vi "3.1-4.7.1-Act Client.vi"() -> ()   [LabVIEW 2010]
doc: "This is the act client, which should send hellos and wait for data. if it receives no data (times out) it continues sending hellos. if it fails in any other way, it closes the UDP connection and starts up a new one. The act control data type is strange because it contains a variant which is either joystick data or arbitratable data. an enumeration controls how it should be interpreted."
uses:
  4-High Neurons/4.0-Super Heart Beat.ctl
  4-High Neurons/4.1-Act Control Typedef.ctl
  4-High Neurons/4.1.0-Datatype Typedef.ctl
  4-High Neurons/4.1.1-Act Joystick.ctl
  4-High Neurons/4.1.2-Act Neuron TD.ctl
  3.0-Global.vi
panel:
  out "Super Heart Beat":T1
  out "Error":errorcluster
  in  "stop":bool
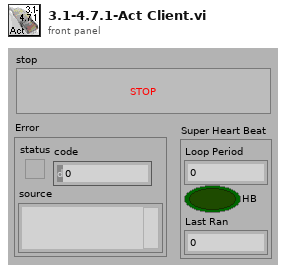
[diagram p1: front panel]
types:
  T1 = typedef "4.0-Super Heart Beat.ctl" = cluster{"Loop Period":u32, "HB":bool, "Last Ran":u32}
  T2 = typedef "4.1.1-Act Joystick.ctl" = cluster{"Trig":bool, "2":bool, "3":bool, "4":bool, "5":bool, "6":bool, "7":bool, "8":bool, "9":bool, "10":bool, "11":bool, "Pitch":i32, "Ang":bool[], "Wheel":dbl, "Roll":i32, "Yaw":i32, "Left":i32, "Right":i32}
  T3 = typedef "4.1.2-Act Neuron TD.ctl" = cluster{"Speed By Path":dbl[]}
  T4 = typedef "4.1-Act Control Typedef.ctl" = cluster{"4.1.0 Data":variant, "Type of Data":T5, "E-Stop":bool, "Restart":bool, "New IP":bool, "Begin":bool, "Time":i32, "Shutdown":bool}
  T5 = typedef "4.1.0-Datatype Typedef.ctl" = enum16{"4.1.0-Empty Data", "4.1.1-Joystick Data", "4.1.2-Behavioral Data"}
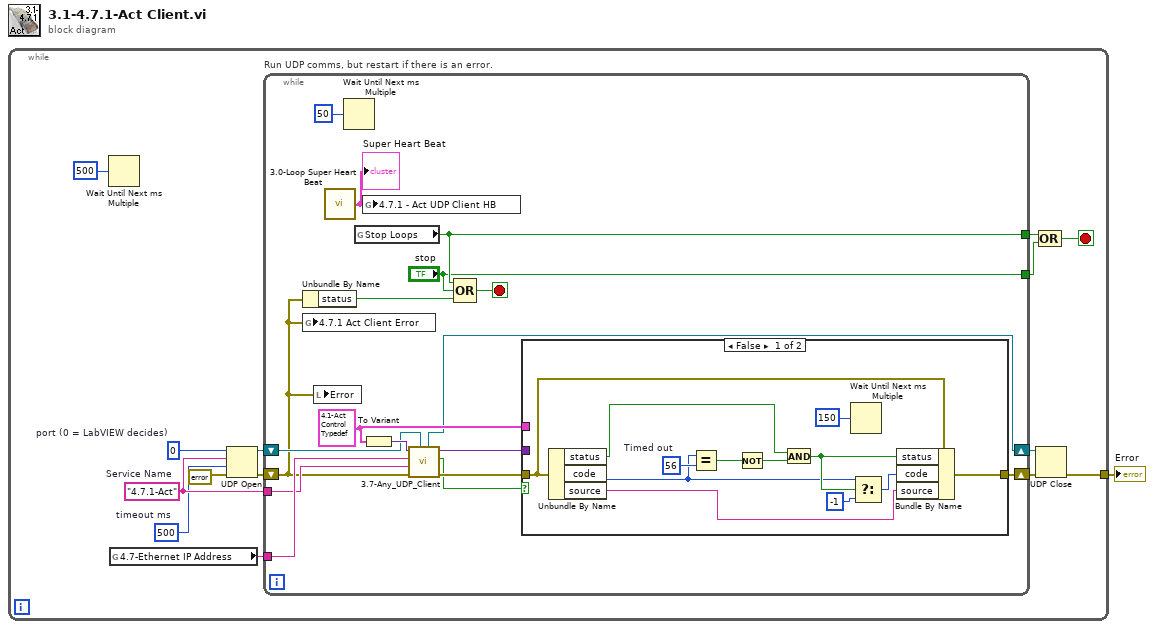
[diagram p0: block diagram]
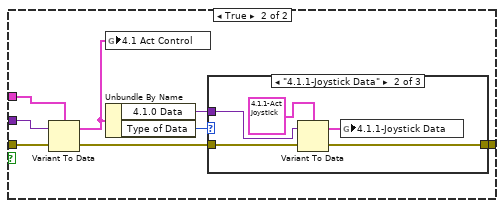
[diagram p2: hidden frame]
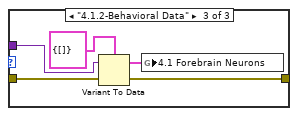
[diagram p4: hidden frame]
diagram:
  n1 = while {
    tunnel: [w3] -> w1
    stop <- w13 stop-if-true
    w6 = 500  # timeout ms
    w8 = u16 0  # port (0 = LabVIEW decides)
    w7 = "4.7.1-Act"  # Service Name
    n2 = Wait Until Next ms Multiple(millisecond multiple=u32 500) -> ()  [unwired: 1 out]
    n3 = global read "3.0-Global.vi" "4.7-Ethernet IP Address"() -> (w5:string)
    n4 = UDP Open(8:errorcluster {"status"=FALSE, "code"=0, "source"=""} ("error in (no error)"), 9:w6, 10:w7, 11:w8) -> (port=w12:refnum<k16>, 0:w10:errorcluster)  [unwired: 1 in, 1 out]
    n5 = while "Run UDP comms, but restart if there is an error." {
      tunnel: w7 -> [w29]
      tunnel: w5 -> [w30]
      tunnel: [w25] -> w15
      tunnel: ["stop"] -> w14
      shift-right: [w21] -> w11
      shift-left: w12 -> [w22]
      shift-right: [w20] -> w9
      shift-left: w10 -> [w17]
      stop <- w32 stop-if-true
      w26 = T4 {"4.1.0 Data"=variant, "Type of Data"=enum."4.1.1-Joystick Data", "E-Stop"=FALSE, "Restart"=FALSE, "New IP"=FALSE, "Begin"=FALSE, "Time"=0, "Shutdown"=FALSE} ("4.1 Act Control")
      n6 = Unbundle By Name(w17) -> ("status"=w23:bool)
      n7 = global write "3.0-Global.vi" "4.7.1 Act Client Error"(w17) -> ()
      n8 = local write "Error"(w17) -> ()
      n9 = call "3.0-Loop Super Heart Beat.vi"() -> ("Super Heart Beat"=w16:T1)
      "Super Heart Beat" <- w16
      n10 = Wait Until Next ms Multiple(millisecond multiple=u32 50) -> ()  [unwired: 1 out]
      n11 = global read "3.0-Global.vi" "Stop Loops"() -> (w25:bool)
      n12 = global write "3.0-Global.vi" "4.7.1 - Act UDP Client HB"(w16) -> ()
      n13 = To Variant(anything=w26) -> (Variant=w28:variant)
      n14 = call "3.7-Any_UDP_Client.vi"("Port In"=w22, "error In"=w17, "Service Name"=w29, "IP Address"=w30, "DataTypeIn"=w28) -> ("Error Out"=w19:errorcluster, "Check Passed"=w18:bool, "DataOut"=w27:variant, "Port out"=w21:refnum<k16>)  [unwired: 3 in]
      n15 = Compound Arithmetic op=OR(w25, "stop", w23) -> (w32:bool)
      n16 = case shown="False" w18 {
        tunnel: w27 -> [_ w52]
        tunnel: w26 -> [_ w51]
        tunnel: w19 -> [w44 w47]
        tunnel: [w43 w46] -> w20
        frame False {
          w42 = 56  # Timed out
          n17 = Unbundle By Name(w44) -> ("status"=w39:bool, "code"=w37:i32, "source"=w34:string)
          n18 = Equal?(x=w37, y=w42) -> (x = y?=w41:bool)
          n19 = Not(x=w41) -> (.not. x?=w40:bool)
          n20 = And(x=w39, y=w40) -> (x .and. y?=w38:bool)
          n21 = Wait Until Next ms Multiple(millisecond multiple=u32 150) -> ()  [unwired: 1 out]
          n22 = Select(t=w37, s=w38, f=-1) -> (s? t:f=w35:i32)
          n23 = Bundle By Name(cluster=w44, "status"=w38, "code"=w35, "source"=w34) -> (w43:errorcluster)
        }
        frame True {
          n24 = Variant To Data(error in=w47, Variant=w52, type=w51) -> (error out=w48:errorcluster, data=w45:T4)
          n25 = global write "3.0-Global.vi" "4.1 Act Control"(w45) -> ()
          n26 = Unbundle By Name(w45) -> ("4.1.0 Data"=w50:variant, "Type of Data"=w49:T5)
          n27 = case shown="\"4.1.1-Joystick Data\"" w49 {
            tunnel: w50 -> [_ w56 w59]
            tunnel: w48 -> [w53 w55 w61]
            tunnel: [w53 w54 w60] -> w46
            frame "4.1.0-Empty Data", Default {
            }
            frame "4.1.1-Joystick Data" {
              n28 = Variant To Data(error in=w55, Variant=w56, type=T2 {"Trig"=FALSE, "2"=FALSE, "3"=FALSE, "4"=FALSE, "5"=FALSE, "6"=FALSE, "7"=FALSE, "8"=FALSE, "9"=FALSE, "10"=FALSE, "11"=FALSE, "Pitch"=0, "Ang"=[], "Wheel"=0.0, "Roll"=0, "Yaw"=0, "Left"=0, "Right"=0} ("Saitek Controler")) -> (error out=w54:errorcluster, data=w57:T2)
              n29 = global write "3.0-Global.vi" "4.1.1-Joystick Data"(w57) -> ()
            }
            frame "4.1.2-Behavioral Data" {
              n30 = Variant To Data(error in=w61, Variant=w59, type=T3 {"Speed By Path"=[]} ("Forebrain Act Neurons")) -> (error out=w60:errorcluster, data=w62:T3)
              n31 = global write "3.0-Global.vi" "4.1 Forebrain Neurons"(w62) -> ()
            }
          }
        }
      }
    }
    n32 = UDP Close(connection ID=w11, 8:w9) -> (error out=w3:errorcluster)  [unwired: 1 out]
    n33 = Compound Arithmetic op=OR(w15, w14) -> (w13:bool)
  }
  "Error" <- w1
